vi "SwrvLinAlg Drive v2.vi"(6 "Auto Controls":bool, 8 "Robot-Centric":bool, 9 "Z":dbl(knob) scale=1.0..-1.0, 10 "Y":dbl(slide) scale=1.0..-1.0, 11 "X":dbl(slide) scale=-1.0..1.0) -> ()   [LabVIEW 2017]
uses:
  SwrvLinAlg Wheel Core Debug Outputs.ctl
  SwrvLinAlg XY Relative to Robot.vi
  SwrvLinAlg Full Spin Logic.vi
  <vilib>/Analysis/baseanly.llb/A x B.vi
  <vilib>/Analysis/baseanly.llb/A x Vector.vi
  Robot Global Data.vi
  <vilib>/Rock Robotics/Network Tables/NT Read Value.vi
  <vilib>/Rock Robotics/Network Tables/NT Read Number.vi
  Public/Documents/Cross The Road Electronics/Phoenix-LabVIEW/Motor Controller/CTRE_Phoenix_MotorControl_RefNumRegistryGet.vi
  Public/Documents/Cross The Road Electronics/Phoenix-LabVIEW/Motor Controller/CTRE_Phoenix_MotorController_Get_Enhanced.vi
  Public/Documents/Cross The Road Electronics/Phoenix-LabVIEW/Motor Controller/Get/CTRE_Phoenix_MotorController_GetPulseWidthAll.vi
  Convert Encoder to Angle v2.vi
  Convert Angle to Encoder v2.vi
  <vilib>/Rock Robotics/WPI/ThirdParty/Phoenix-LabVIEW/Motor Controller/CTRE_Phoenix_MotorControl_Set.vi
  <vilib>/Rock Robotics/Network Tables/NT Write Boolean Array.vi
panel:
  out "Controller":cluster{"X":dbl, "X":dbl, "X":dbl}(graph)
  out "Gyro":dbl(graph)
  out "BR Sent":dbl(graph)
  out "BL Sent":dbl(graph)
  out "FR Sent":dbl(graph)
  out "FL Sent":dbl(graph)
  out "BR Position":dbl(graph)
  out "BL Position":dbl(graph)
  out "FR Position":dbl(graph)
  out "FL Position":dbl(graph)
  out "Back Right":T1
  out "Back Left":T1
  out "Front Right":T1
  out "Front Left":T1
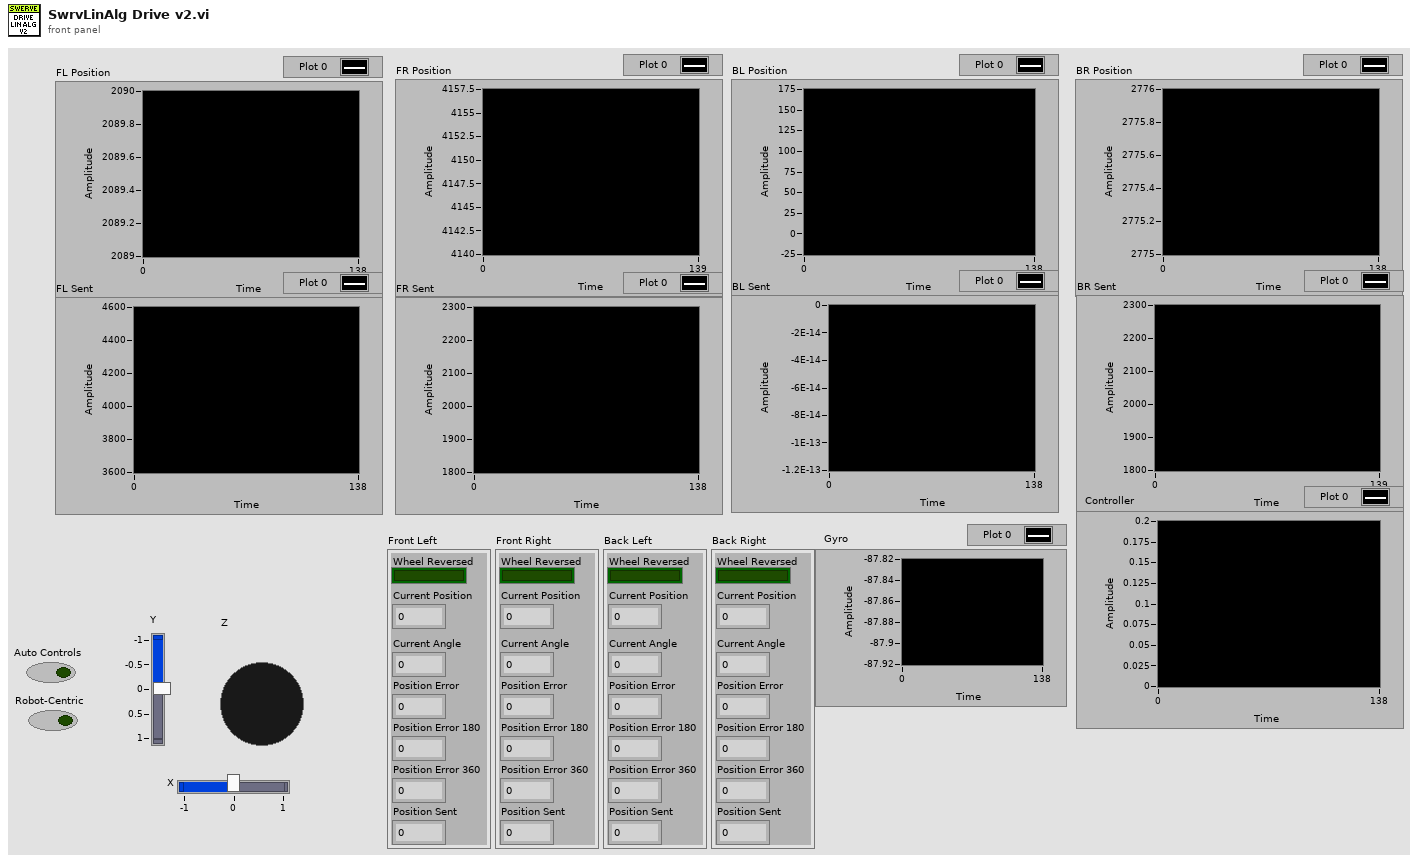
[diagram p1: front panel]
types:
  T1 = typedef "SwrvLinAlg Wheel Core Debug Outputs.ctl" = cluster{"Wheel Reversed":bool, "Current Angle":dbl, "Position Error":dbl, "Position Error 180":dbl, "Position Error 360":dbl, "Position Sent":dbl, "Current Position":dbl}
  T2 = enum16{"Front Left", "Front Right", "Back Left", "Back Right"}
  T3 = typedef "WPI_MotorControlDeviceRef.ctl" = cluster{"DeviceStatus":errorcluster, "Type":T4, "PWM":cluster{"PWM Channel":T5, "DeadBand":T6}, "CAN":cluster{"Device Number":u8, "SetOutput VI Ref":variant, "GetOutput VI Ref":variant, "Enable VI Ref":variant, "Disable VI Ref":variant, "Data":variant}, "Invert":bool, "DIO PWM":cluster{"PWM \"Enable\" Channel":T5, "DIOChannel":T7, "PWM Rate":dbl}}
  T4 = typedef "WPI_MotorControlType.ctl" = enum16{"PWM", "CAN", "DIO PWM"}
  T5 = typedef "FPGA_DIOPWMChannel.ctl" = enum8{"PWM 0", "PWM 1", "PWM 2", "PWM 3", "PWM 4", "PWM 5", "PWM 6", "PWM 7", "PWM 8", "PWM 9", "PWM MXP 0", "PWM MXP 1", "PWM MXP 2", "PWM MXP 3", "PWM MXP 4", "PWM MXP 5", "PWM MXP 6", "PWM MXP 7", "PWM MXP 8", "PWM MXP 9", "Invalid"}
  T6 = typedef "WPI_PWMDeadband.ctl" = cluster{"Name":string, "maxPositivePwm":i32, "minPositivePwm":i32, "centerPwm":i32, "maxNegativePwm":i32, "minNegativePwm":i32, "angularRange":u16}
  T7 = typedef "FPGA_DIOChannel.ctl" = enum8{"DIO 0", "DIO 1", "DIO 2", "DIO 3", "DIO 4", "DIO 5", "DIO 6", "DIO 7", "DIO 8", "DIO 9", "DIO MXP 0", "DIO MXP 1", "DIO MXP 2", "DIO MXP 3", "DIO MXP 4", "DIO MXP 5", "DIO MXP 6", "DIO MXP 7", "DIO MXP 8", "DIO MXP 9", "DIO MXP 10", "DIO MXP 11", "DIO MXP 12", "DIO MXP 13", "DIO MXP 14", "DIO MXP 15", "SPI Port CS1", "SPI Port CS2", "SPI Port CS3", "SPI Port MISO", "SPI Port MOSI", "Invalid"}
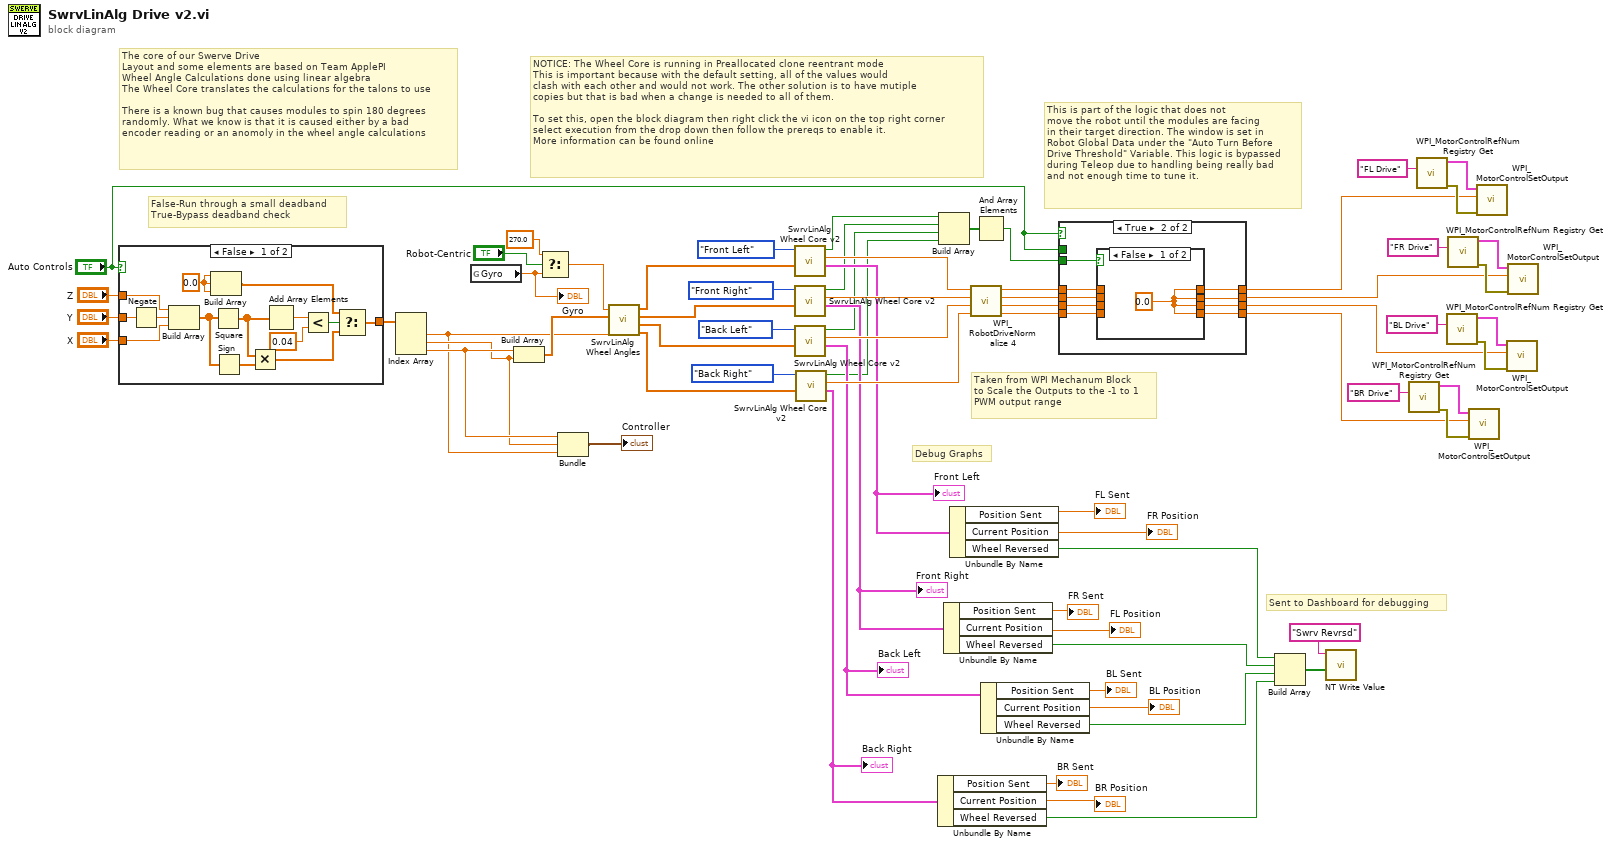
[diagram p0: block diagram]
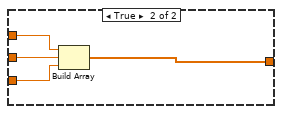
[diagram p4: hidden frame]
diagram:
  # "NOTICE: The Wheel Core is running in Preallocated clone reentrant mode\nThis is important because with the default setting, all of the values would\nclash with each other and would not work. The other solution is to have mutiple\ncopies but that is bad when a change is needed to all of them.\n\nTo set this, open the block diagram then right click the vi icon on the top right corner\nselect execution from the drop down then follow the prereqs to enable it.\nMore information can be found online"
  # "Sent to Dashboard for debugging"
  # "Debug Graphs"
  # "This is part of the logic that does not\nmove the robot until the modules are facing\nin their target direction. The window is set in\nRobot Global Data under the \"Auto Turn Before\nDrive Threshold\" Variable. This logic is bypassed\nduring Teleop due to handling being really bad\nand not enough time to tune it."
  # "Taken from WPI Mechanum Block\nto Scale the Outputs to the -1 to 1\nPWM output range"
  # "The core of our Swerve Drive\nLayout and some elements are based on Team ApplePI\nWheel Angle Calculations done using linear algebra\nThe Wheel Core translates the calculations for the talons to use\n\nThere is a known bug that causes modules to spin 180 degrees\nrandomly. What we know is that it is caused either by a bad\nencoder reading or an anomoly in the wheel angle calculations"
  # "False-Run through a small deadband\nTrue-Bypass deadband check"
  n1 = case shown="False" "Auto Controls" {
    tunnel: "Y" -> [w81 w87]
    tunnel: "X" -> [w75 w88]
    tunnel: "Z" -> [w71 w85]
    tunnel: [w72 w86] -> w67
    frame False {
      w79 = 0.0 ("element")
      n2 = Negate(x=w81) -> (-x=w74:dbl)
      n3 = Build Array(w71, w74, w75) -> (w78:dbl[])
      n4 = Build Array(w79, w79, w79) -> (w80:dbl[])
      n5 = Square(x=w78) -> (x^2=w76:dbl[])
      n6 = Sign(1:w78) -> (0:w77:dbl[])
      n7 = Multiply(x=w76, y=w77) -> (x*y=w73:dbl[])
      n8 = Add Array Elements(numeric array=w76) -> (sum=w84:dbl)
      n9 = Less?(x=w84, y=0.04 ("x")) -> (x < y?=w82:bool)
      n10 = Select(t=w80, s=w82, f=w73) -> (s? t:f=w72:dbl[])
    }
    frame True {
      n11 = Build Array(w85, w87, w88) -> (w86:dbl[])
    }
  }
  n12 = Index Array(array=w67) -> (element #1=w31:dbl, element #2=w33:dbl, element #3=w34:dbl)  [unwired: 3 in]
  n13 = global read "Robot Global Data.vi" "Gyro"() -> (w30:dbl)
  "Gyro" <- w30
  n14 = Build Array(w34, w33) -> (w35:dbl[])
  n15 = Select(t=270.0, s="Robot-Centric", f=w30) -> (s? t:f=w65:dbl)
  n16 = Bundle("X"=w34, "X"=w33, "X"=w31) -> (→"Controller":cluster{"X":dbl, "X":dbl, "X":dbl})  [unwired: 1 in]
  n17 = call "SwrvLinAlg Wheel Angles.vi"("Rotate In"=w31, "x,y movement vector"=w35, "Theta"=w65) -> ("BR Final"=w16:dbl[], "BL Final"=w17:dbl[], "FR Final"=w18:dbl[], "FL Final"=w19:dbl[])  [unwired: 5 in]
  n18 = call "SwrvLinAlg Wheel Core v2.vi"("XY Input"=w19, "Wheel"=T2."Front Left") -> ("Debug Outputs"=w39:T1, "Drive Output"=w47:dbl, "In Range?"=w12:bool)  [unwired: 7 in]
  "Front Left" <- w39
  n19 = call "SwrvLinAlg Wheel Core v2.vi"("XY Input"=w18, "Wheel"=T2."Front Right") -> ("Debug Outputs"=w38:T1, "Drive Output"=w44:dbl, "In Range?"=w13:bool)  [unwired: 7 in]
  "Front Right" <- w38
  n20 = call "SwrvLinAlg Wheel Core v2.vi"("XY Input"=w17, "Wheel"=T2."Back Left") -> ("Debug Outputs"=w43:T1, "Drive Output"=w45:dbl, "In Range?"=w14:bool)  [unwired: 7 in]
  "Back Left" <- w43
  n21 = call "SwrvLinAlg Wheel Core v2.vi"("XY Input"=w16, "Wheel"=T2."Back Right") -> ("Debug Outputs"=w42:T1, "Drive Output"=w46:dbl, "In Range?"=w15:bool)  [unwired: 7 in]
  "Back Right" <- w42
  n22 = Unbundle By Name(w42) -> ("Position Sent"=→"BR Sent":dbl, "Current Position"=→"BR Position":dbl, "Wheel Reversed"=w20:bool)
  n23 = Build Array(w12, w13, w14, w15) -> (w11:bool[])
  n24 = Unbundle By Name(w38) -> ("Position Sent"=→"FR Sent":dbl, "Current Position"=→"FL Position":dbl, "Wheel Reversed"=w22:bool)
  n25 = Unbundle By Name(w39) -> ("Position Sent"=→"FL Sent":dbl, "Current Position"=→"FR Position":dbl, "Wheel Reversed"=w24:bool)
  n26 = call <vilib>:"WPI_RobotDriveNormalize 4.vi"("D"=w46, "C"=w45, "B"=w44, "A"=w47) -> ("D'"=w4:dbl, "C'"=w6:dbl, "B'"=w7:dbl, "A'"=w9:dbl)
  n27 = And Array Elements(Boolean array=w11) -> (logical AND=w2:bool)
  n28 = Unbundle By Name(w43) -> ("Position Sent"=→"BL Sent":dbl, "Current Position"=→"BL Position":dbl, "Wheel Reversed"=w21:bool)
  n29 = case shown="True" "Auto Controls" {
    tunnel: [w92 w100] -> w10
    tunnel: w9 -> [w92 w99]
    tunnel: [w91 w97] -> w8
    tunnel: w7 -> [w91 w98]
    tunnel: w6 -> [w90 w96]
    tunnel: [w90 w95] -> w5
    tunnel: w4 -> [w89 w94]
    tunnel: [w89 w93] -> w3
    tunnel: w2 -> [_ w101]
    tunnel: "Auto Controls" -> [_ _]
    frame False {
    }
    frame True {
      n30 = case shown="False" w101 {
        tunnel: [w102 w106] -> w100
        tunnel: w99 -> [_ w106]
        tunnel: w98 -> [_ w105]
        tunnel: [w102 w105] -> w97
        tunnel: w96 -> [_ w104]
        tunnel: [w102 w104] -> w95
        tunnel: w94 -> [_ w103]
        tunnel: [w102 w103] -> w93
        frame False {
          w102 = 0.0 ("A'")
        }
        frame True {
        }
      }
    }
  }
  n31 = Build Array(w24, w22, w21, w20) -> (w23:bool[])
  n32 = call-poly <vilib>:"NT Write Value.vi"("Boolean Array"=w23, "Name"="Swrv Revrsd") -> ()  [unwired: 9 in, 1 out]
  n33 = call <vilib>:"WPI_MotorControlRefNum Registry Get.vi"("refnum name"="BR Drive") -> ("error out"=w52:errorcluster, "MotorControlDevRef"=w54:T3)  [unwired: 9 in]
  n34 = call <vilib>:"WPI_MotorControlRefNum Registry Get.vi"("refnum name"="FL Drive") -> ("error out"=w61:errorcluster, "MotorControlDevRef"=w63:T3)  [unwired: 9 in]
  n35 = call <vilib>:"WPI_MotorControlRefNum Registry Get.vi"("refnum name"="BL Drive") -> ("error out"=w55:errorcluster, "MotorControlDevRef"=w57:T3)  [unwired: 9 in]
  n36 = call <vilib>:"WPI_MotorControlRefNum Registry Get.vi"("refnum name"="FR Drive") -> ("error out"=w58:errorcluster, "MotorControlDevRef"=w60:T3)  [unwired: 9 in]
  n37 = call <vilib>:"WPI_MotorControlSetOutput.vi"("error in (no error)"=w52, "Output"=w3, "MotorControlDevRef"=w54) -> ()  [unwired: 6 in, 3 out]
  n38 = call <vilib>:"WPI_MotorControlSetOutput.vi"("error in (no error)"=w61, "Output"=w10, "MotorControlDevRef"=w63) -> ()  [unwired: 6 in, 3 out]
  n39 = call <vilib>:"WPI_MotorControlSetOutput.vi"("error in (no error)"=w55, "Output"=w5, "MotorControlDevRef"=w57) -> ()  [unwired: 6 in, 3 out]
  n40 = call <vilib>:"WPI_MotorControlSetOutput.vi"("error in (no error)"=w58, "Output"=w8, "MotorControlDevRef"=w60) -> ()  [unwired: 6 in, 3 out]
